vi "Append Element to Array (by ref) [U32].vi"(8 "Error In":errorcluster, 9 "New Element":u32, 11 "Array in":refnum<vi>) -> (0 "Error Out":errorcluster, 1 "Array w New Element":u32[](array[numeric]), 3 "Array out":refnum<vi>)   [LabVIEW 2021, in "Arrays.lvlib"]
doc: "Appends an element to a U32 array control using its reference."
uses:
  Arrays.lvlib
panel:
  # "see the AlliGator License on the block diagram (Ctrl+E or Window:Show Block Diagram)"
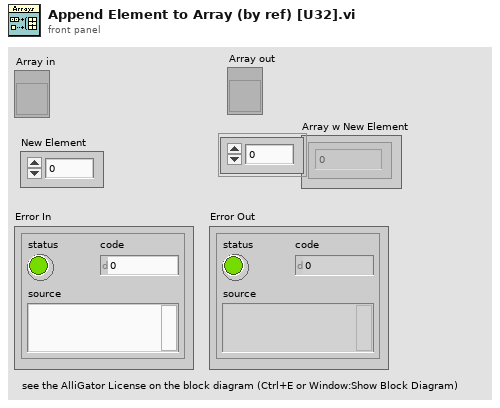
[diagram p1: front panel]
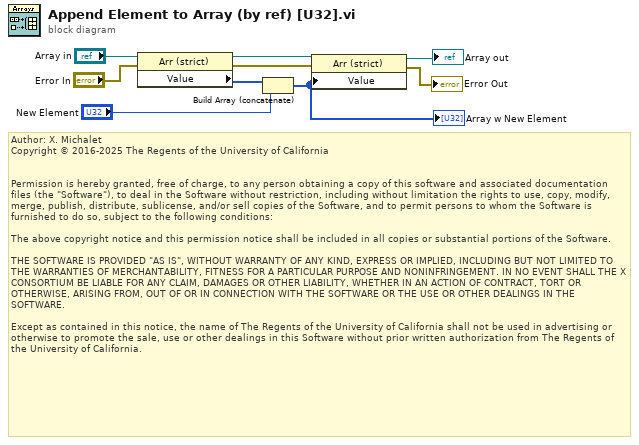
[diagram p0: block diagram]
diagram:
  # "Author: X. Michalet\nCopyright © 2016-2025 The Regents of the University of California\n \n\nPermission is hereby granted, free of charge, to any person obtaining a copy of this software and associated documentation files (the \"Software\"), to deal in the Software without restriction, including without limitation the rights to use, copy, modify, merge, publish, distribute, sublicense, and/or sell copies of the Software, and to permit persons to whom the Software is furnished to do so, subject to the following conditions:\n\nThe above copyright notice and this permission notice shall be included in all copies or substantial portions of the Software.\n\nTHE SOFTWARE IS PROVIDED \"AS IS\", WITHOUT WARRANTY OF ANY KIND, EXPRESS OR IMPLIED, INCLUDING BUT NOT LIMITED TO THE WARRANTIES OF MERCHANTABILITY, FITNESS FOR A PARTICULAR PURPOSE AND NONINFRINGEMENT. IN NO EVENT SHALL THE X CONSORTIUM BE LIABLE FOR ANY CLAIM, DAMAGES OR OTHER LIABILITY, WHETHER IN AN ACTION OF CONTRACT, TORT OR OTHERWISE, ARISING FROM, OUT OF OR IN CONNECTION WITH THE SOFTWARE OR THE USE OR OTHER DEALINGS IN THE SOFTWARE.\n\nExcept as contained in this notice, the name of The Regents of the University of California shall not be used in advertising or otherwise to promote the sale, use or other dealings in this Software without prior written authorization from The Regents of the University of California."
  n1 = property class="Arr (strict)"(reference="Array in", error in="Error In") -> (reference out=w8:refnum<vi>, error out=w4:errorcluster, "Value"=w7:u32[])
  n2 = Build Array (concatenate)(w7, "New Element") -> (w1:u32[])
  "Array w New Element" <- w1
  n3 = property class="Arr (strict)"(reference=w8, error in=w4, "Value"=w1) -> (reference out=→"Array out":refnum<vi>, error out=→"Error Out":errorcluster)
